vi "Find Topmost Partial Match.vi"(10 "Name":string, 11 "Tree":variant) -> (1 "Found?":bool, 2 "Match":variant, 3 "Node Name":string)   [LabVIEW 2019, in "Tree.lvclass"]
uses:
  Tree.lvclass
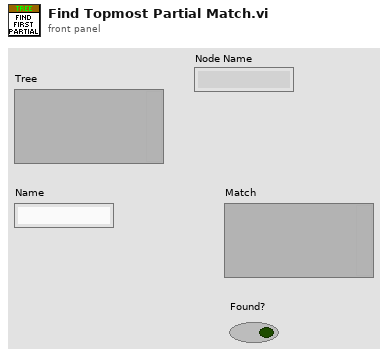
[diagram p1: front panel]
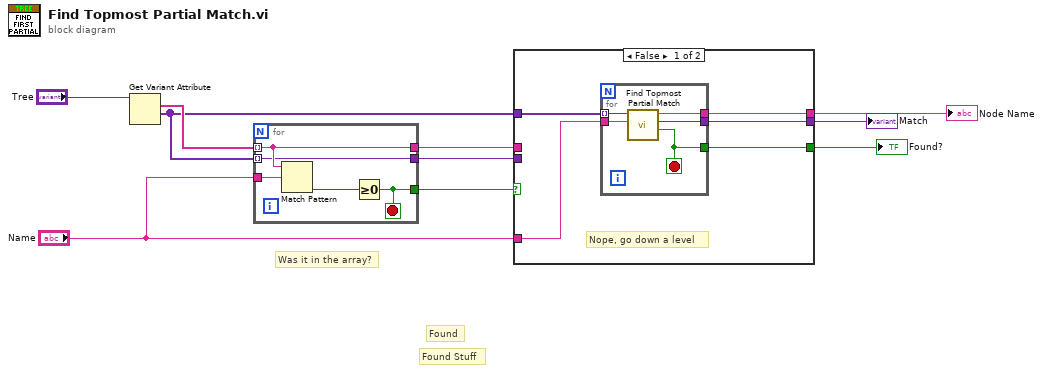
[diagram p0: block diagram]
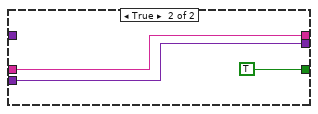
[diagram p2: hidden frame]
diagram:
  # "Was it in the array?"
  # "Found Stuff"
  # "Found"
  n1 = Get Variant Attribute(Variant="Tree") -> (names=w7:string[], values=w6:variant[])  [unwired: 3 in, 2 out]
  n2 = for {
    tunnel: w7 -> [w13] mode=indexing
    tunnel: "Name" -> [w15]
    tunnel: [w13] -> w3
    tunnel: [w12] -> w5
    tunnel: w6 -> [w11] mode=indexing
    tunnel: [w11] -> w2
    stop <- w12 stop-if-true
    n3 = Match Pattern(string=w13, regular expression=w15) -> (offset past match=w14:i32)  [unwired: 1 in, 3 out]
    n4 = Greater Or Equal To 0?(x=w14) -> (x >= 0?=w12:bool)
  }
  n5 = case shown="False" w5 {
    tunnel: "Name" -> [w20 _]
    tunnel: w6 -> [w17 _]
    tunnel: [w19 w27] -> w9
    tunnel: [w18 TRUE ("Found?")] -> w8
    tunnel: w3 -> [_ w26]
    tunnel: w2 -> [_ w27]
    tunnel: [w16 w26] -> w1
    frame False {
      # "Nope, go down a level"
      n6 = for {
        tunnel: w17 -> [w25] mode=indexing
        tunnel: w20 -> [w23]
        tunnel: [w24] -> w19
        tunnel: [w22] -> w18
        tunnel: [w21] -> w16
        stop <- w22 stop-if-true
        n7 = call "Find Topmost Partial Match.vi"("Name"=w23, "Tree"=w25) -> ("Found?"=w22:bool, "Match"=w24:variant, "Node Name"=w21:string)  [unwired: 7 in]
      }
    }
    frame True {
    }
  }
  "Found?" <- w8
  "Match" <- w9
  "Node Name" <- w1
